vi "Check Start.vi"(8 "error in":errorcluster, 11 "Error Stop?":bool) -> (0 "error out":errorcluster, 2 "Message":string)   [LabVIEW 2021]
uses:
  Global Variables/FPGA GV.vi
  <vilib>/Utility/error.llb/Error Cluster From Error Code.vi
  <vilib>/rvi/errors/niLvFpgaAdjustHostInterfaceError.vi
  Global Variables/RT GV.vi
  <vilib>/rvi/interface/nirviReadWriteControl/nirviReadWriteControl.xnode
  NiFpgaLv.dll
  <vilib>/rvi/interface/Simulation/niFpgaSimulationCallBeginRW.vi
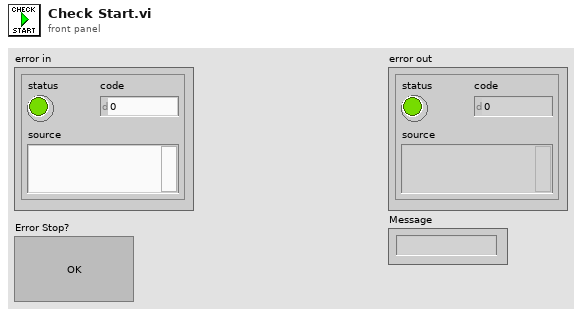
[diagram p1: front panel]
types:
  T1 = cluster{"Machine_ON":bool, "E_stop ":bool, "SW_Pressure":bool, "SW_Start ":bool, "SW_Reset":bool, "SW_Stop":bool, "SW_Door":bool, "Buffer 1":bool, "Buffer 2":bool, "RS_Index_Stopper _Rear":bool, "RS_Singling_Rear":bool, "PES_Index_Pallet_Sensor":bool, "PES_Index_Output_Part Sensor":bool, "Buffer 3":bool, "SW_Cutting_Station_Door":bool, "ICS_BF_Pump_CNVR_Full_1":bool, "ICS_BF_Pump_CNVR_Full_2":bool, "ICS_BF_Pump_CNVR_Full_3":bool, "ICS_BF_Pump_CNVR_Full_4":bool, "PES_PC_Pump Presence_1":bool, "PES_PC_Pump Presence_2":bool, "PES_PC_Pump Presence_3":bool, "PES_PC_Pump Presence_4":bool, "RS_Pick_Place_Vertical":bool, "Buffer 4":bool, "PES_TF_Low_Level":bool, "RS_Cutting_Rear 1":bool, "RS_Cutting_Rear 2":bool, "RS_Cutting_Rear 3":bool, "RS_Cutting_Rear 4":bool, "RS_Cutting_Forward_Rear":bool, "Buffer 10":bool}
  T2 = cluster{"RS_Agitatator_1_Rear ":bool, "Buffer 1 ":bool, "RS_TF_Gating CYL_Rear":bool, "RS_Insertion_1_Rear":bool, "RS_Insertion_1_Front":bool, "RS_Insertion _2_Rear":bool, "RS_Insertion _2_Front":bool, "RS_Insertion _3_Rear":bool, "RS_Insertion _3_Front":bool, "RS_Insertion _4_Rear":bool, "RS_Insertion _4_Front":bool, "RS_Insertion_Clamp_CYL":bool, "RS_Cutting_Rear":bool, "RS_Clamping_Rear":bool, "RS_Measurement_Front":bool, "RS_Measurement_Rear":bool, "Buffer 3":bool, "Buffer 4":bool, "Buffer 5":bool, "RS_Rejection_1_Rear":bool, "RS_Rejection_2_Rear":bool, "RS_Rejection_3_Rear":bool, "RS_Rejection_4_Rear":bool, "Buffer 6 ":bool, "Buffer 7 ":bool, "LS_Rotary_P&P":bool, "Vaccum Components check":bool, "Buffer 10 ":bool, "Buffer 11 ":bool, "Buffer 12 ":bool, "Buffer 13 ":bool, "Buffer 14":bool}
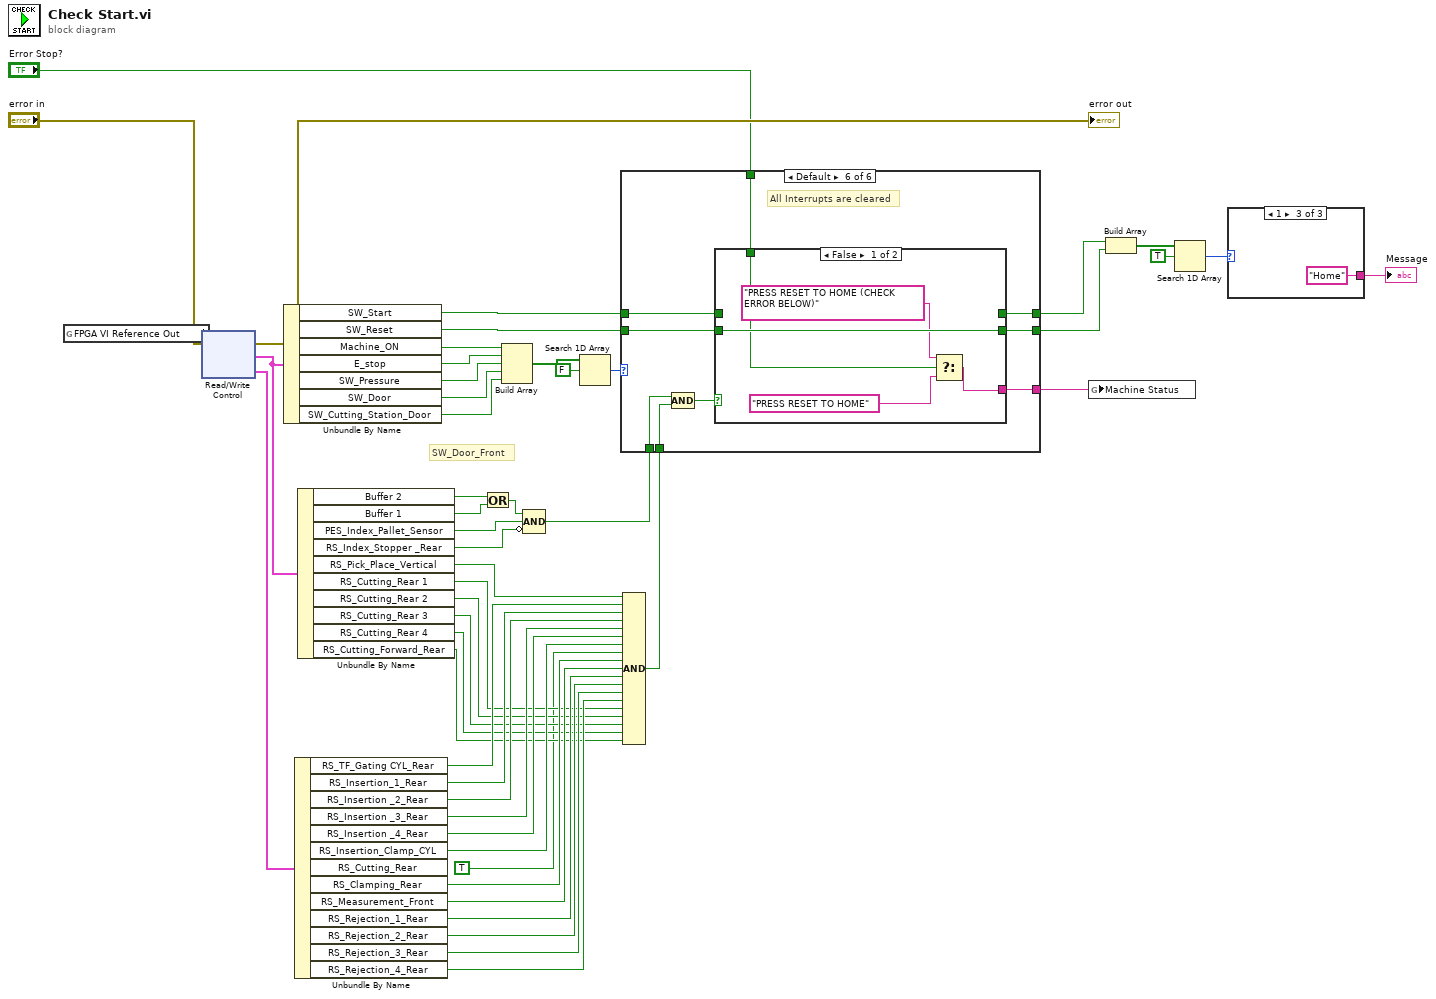
[diagram p0: block diagram]
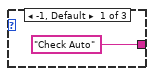
[diagram p2: hidden frame]
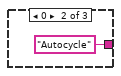
[diagram p3: hidden frame]
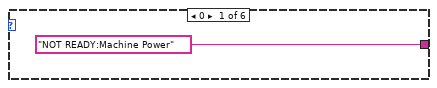
[diagram p4: hidden frame]
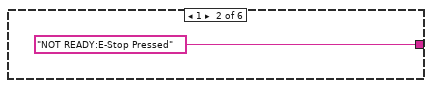
[diagram p5: hidden frame]
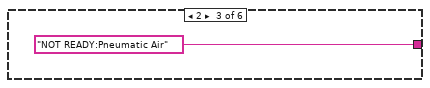
[diagram p6: hidden frame]
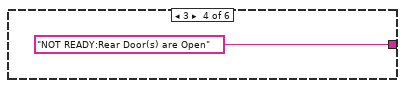
[diagram p7: hidden frame]
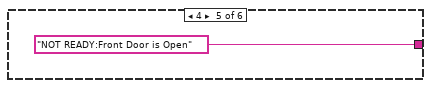
[diagram p8: hidden frame]
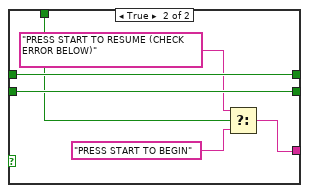
[diagram p9: hidden frame]
diagram:
  # "SW_Door_Front"
  n1 = global read "FPGA GV.vi" "FPGA VI Reference Out"() -> (w47:refnum<k20>)
  n2 = xnode "Read/Write Control"("FPGA VI Reference In"=w47, "error in"="error in") -> ("error out"=→"error out":errorcluster, "DI 1"=w39:T1, "DI 2"=w23:T2)  [unwired: 1 out]
  n3 = Unbundle By Name(w39) -> ("SW_Start"=w21:bool, "SW_Reset"=w40:bool, "Machine_ON"=w46:bool, "E_stop"=w45:bool, "SW_Pressure"=w13:bool, "SW_Door"=w12:bool, "SW_Cutting_Station_Door"=w7:bool)
  n4 = Unbundle By Name(w23) -> ("RS_TF_Gating CYL_Rear"=w25:bool, "RS_Insertion_1_Rear"=w35:bool, "RS_Insertion _2_Rear"=w34:bool, "RS_Insertion _3_Rear"=w33:bool, "RS_Insertion _4_Rear"=w32:bool, "RS_Insertion_Clamp_CYL"=w31:bool, "RS_Clamping_Rear"=w30:bool, "RS_Measurement_Front"=w11:bool, "RS_Rejection_1_Rear"=w29:bool, "RS_Rejection_2_Rear"=w28:bool, "RS_Rejection_3_Rear"=w27:bool, "RS_Rejection_4_Rear"=w26:bool)  [unwired: 1 out]
  n5 = Unbundle By Name(w39) -> ("Buffer 2"=w9:bool, "Buffer 1"=w10:bool, "PES_Index_Pallet_Sensor"=w38:bool, "RS_Index_Stopper _Rear"=w37:bool, "RS_Pick_Place_Vertical"=w24:bool, "RS_Cutting_Rear 1"=w6:bool, "RS_Cutting_Rear 2"=w5:bool, "RS_Cutting_Rear 3"=w4:bool, "RS_Cutting_Rear 4"=w3:bool, "RS_Cutting_Forward_Rear"=w2:bool)
  n6 = Or(x=w9, y=w10) -> (x .or. y?=w8:bool)
  n7 = Build Array(w46, w45, w13, w12, w7) -> (w42:bool[])
  n8 = Compound Arithmetic op=AND(w8, w38, invert w37) -> (w36:bool)
  n9 = Search 1D Array(1D array=w42, element=FALSE) -> (index of element=w44:i32)  [unwired: 1 in]
  n10 = Compound Arithmetic op=AND(w24, w25, w35, w34, w33, w32, w31, TRUE, w30, w11, w29, w28, w27, w26, w6, w5, w4, w3, w2) -> (w22:bool)
  n11 = case shown="Default" w44 {
    tunnel: ["NOT READY:Machine Power" "NOT READY:E-Stop Pressed" "NOT READY:Pneumatic Air" "NOT READY:Rear Door(s) are Open" "NOT READY:Front Door is Open" w63] -> w41
    tunnel: w40 -> [_ _ _ _ _ w58]
    tunnel: w36 -> [_ _ _ _ _ w62]
    tunnel: w22 -> [_ _ _ _ _ w61]
    tunnel: w21 -> [_ _ _ _ _ w59]
    tunnel: [_ _ _ _ _ w57] -> w20
    tunnel: [_ _ _ _ _ w56] -> w19
    tunnel: "Error Stop?" -> [_ _ _ _ _ w55]
    frame 0 {
    }
    frame 1 {
    }
    frame 2 {
    }
    frame 3 {
    }
    frame 4 {
    }
    frame Default {
      # "All Interrupts are cleared"
      n12 = Compound Arithmetic op=AND(w62, w61) -> (w60:bool)
      n13 = case shown="False" w60 {
        tunnel: [w66 w71] -> w63
        tunnel: w59 -> [_ w74]
        tunnel: w58 -> [w68 w73]
        tunnel: [_ w74] -> w57
        tunnel: [w68 w73] -> w56
        tunnel: w55 -> [w64 w70]
        frame False {
          n14 = Select(t="PRESS RESET TO HOME (CHECK ERROR BELOW)", s=w64, f="PRESS RESET TO HOME") -> (s? t:f=w66:string)
        }
        frame True {
          n15 = Select(t="PRESS START TO RESUME (CHECK ERROR BELOW)", s=w70, f="PRESS START TO BEGIN") -> (s? t:f=w71:string)
        }
      }
    }
  }
  n16 = global write "RT GV.vi" "Machine Status"(w41) -> ()
  n17 = Build Array(w20, w19) -> (w17:bool[])
  n18 = Search 1D Array(1D array=w17, element=TRUE) -> (index of element=w16:i32)  [unwired: 1 in]
  n19 = case shown="1" w16 {
    tunnel: ["Check Auto" ("Message") "Autocycle" ("Message") "Home" ("Message")] -> w15
    frame -1, Default {
    }
    frame 0 {
    }
    frame 1 {
    }
  }
  "Message" <- w15
